vi "Send UpDataResult.vi"(7 "Message Priority (Normal)":T2=enum."Normal", 8 "error in (no error)":errorcluster, 9 "Time":dbl, 10 "UpDataResult":T1={"Socket"=-1, "Result"="EXIT", "Value"="", "Limit"={"High"="", "Low"=""}, "Type"="", "StepName"="", "Normal"="", "Unit"=""}, 11 "Message Enqueuer":refnum<class "Message Enqueuer.lvclass">) -> (0 "error out":errorcluster, 3 "Message Enqueuer out":refnum<class "Message Enqueuer.lvclass">)   [LabVIEW 2019, in "UnitTestEngine.lvlib" / "UpDataResult Msg.lvclass"]
doc: "This VI sends the message to an actor."
uses:
  UpDataResult Msg.lvclass
  <vilib>/ActorFramework/Message Enqueuer/Message Enqueuer.lvclass
  <vilib>/ActorFramework/Message Enqueuer/Message Priority.ctl
  C:/Program Files (x86)/National Instruments/LabVIEW 2019/vi.lib/ActorFramework/Message/Message.lvclass
  UpDataResult Msg.lvclass/UpDataResult Msg.ctl
  <vilib>/ActorFramework/Message Enqueuer/Message Enqueuer.lvclass/Message Enqueuer.ctl
  <vilib>/ActorFramework/Message Priority Queue/Priority Enqueue.vi
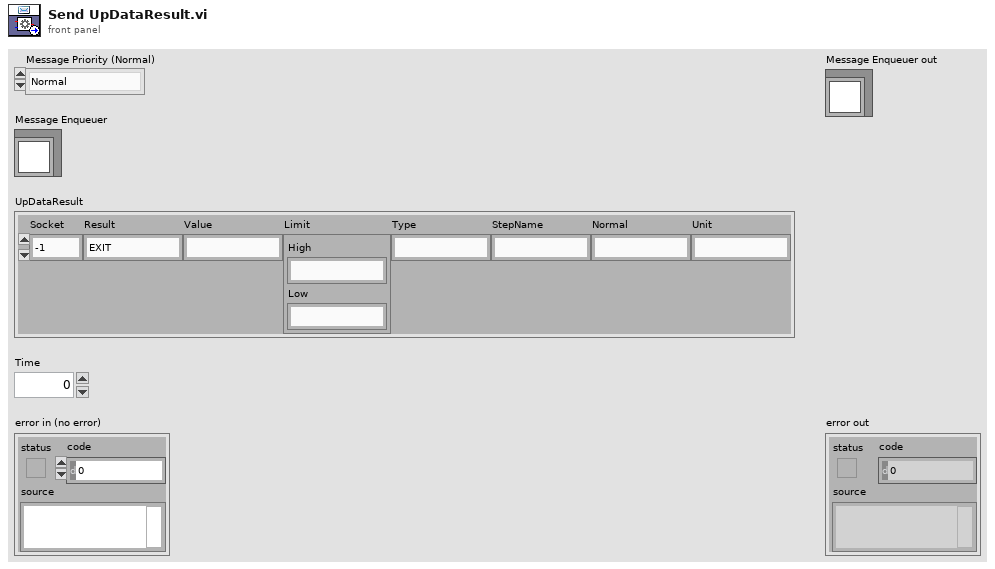
[diagram p1: front panel]
types:
  T1 = cluster{"Socket":i32, "Result":string, "Value":string, "Limit":cluster{"High":string, "Low":string}, "Type":string, "StepName":string, "Normal":string, "Unit":string}
  T2 = typedef "Actor Framework.lvlib/Message Enqueuer.lvclass/Message Priority.ctl" = enum16{"Low", "Normal", "High"}
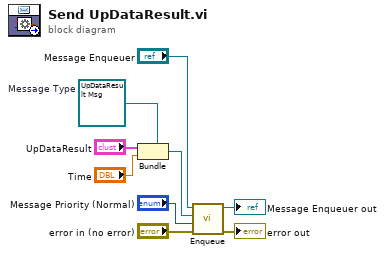
[diagram p0: block diagram]
diagram:
  w3 = refnum<class "UpDataResult Msg.lvclass"> refnum  # Message Type
  n1 = Bundle(cluster=w3, "UpDataResult", "Time") -> (w4:refnum<class "UpDataResult Msg.lvclass">)
  n2 = call <vilib>:"Enqueue.vi"("error in (no error)"="error in (no error)", "Message Priority (Normal)"="Message Priority (Normal)", "Message"=w4, "Message Enqueuer in"="Message Enqueuer") -> ("error out"=→"error out":errorcluster, "Message Enqueuer out"=→"Message Enqueuer out":refnum<class "Message Enqueuer.lvclass">)  [unwired: 6 in]
